vi "3.3-What.vi"() -> ()   [LabVIEW 2010]
uses:
  3.0 Flow Control/3.0 List of Loops.ctl
  4-High Neurons/4.1.2-Act Neuron TD.ctl
  <instrlib>/Hokuyo URG Series/Public/Initialize-Standard.vi
  3.0-Global.vi
  <instrlib>/Hokuyo URG Series/Hokuyo URG Series.lvlib
panel:
  in  "Stop":bool
  out "size(s)":i32
  in  "ID Query?":bool
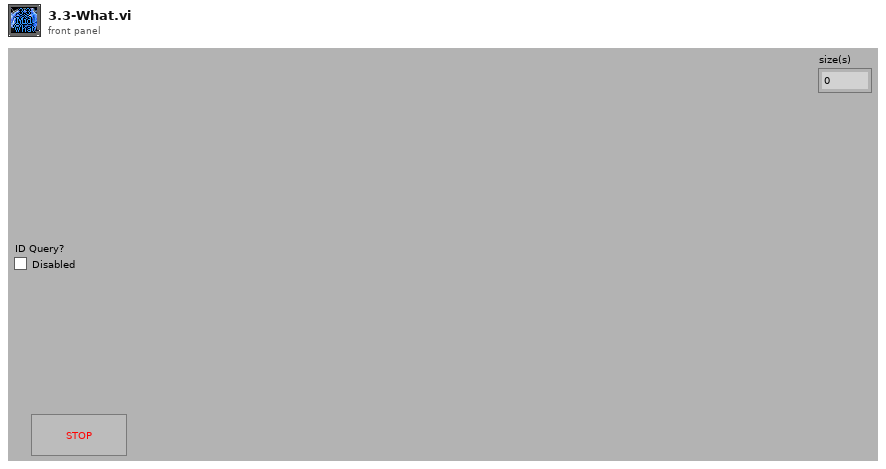
[diagram p1: front panel]
types:
  T1 = typedef "3.0 List of Loops.ctl" = enum16{"3.0 State Update", "3.0 GUI", "3.1 Act", "3.1 4.7.1 Act UDP", "3.1 Joystick", "3.2 Where", "3.2 4.7.2 Where UDP", "3.3 What", "3.3 4.7.3 What UDP", "3.4 How", "3.4 4.7.4 How UDP", "3.5 Limbic", "3.8 TCP", "3.6 Cerebellum"}
  T2 = typedef "4.1.2-Act Neuron TD.ctl" = cluster{"Speed By Path":dbl[]}
  T3 = enum16{"Set Joystick", "Read Joystick", "Set Forebrain", "Read Forebrain", "Set Limbic", "Read Limbic", "Set Cerebellum", "Read Cerebellum", "Set Arbitrated", "Read Arbitrated", "Set LIDAR", "Read LIDAR"}
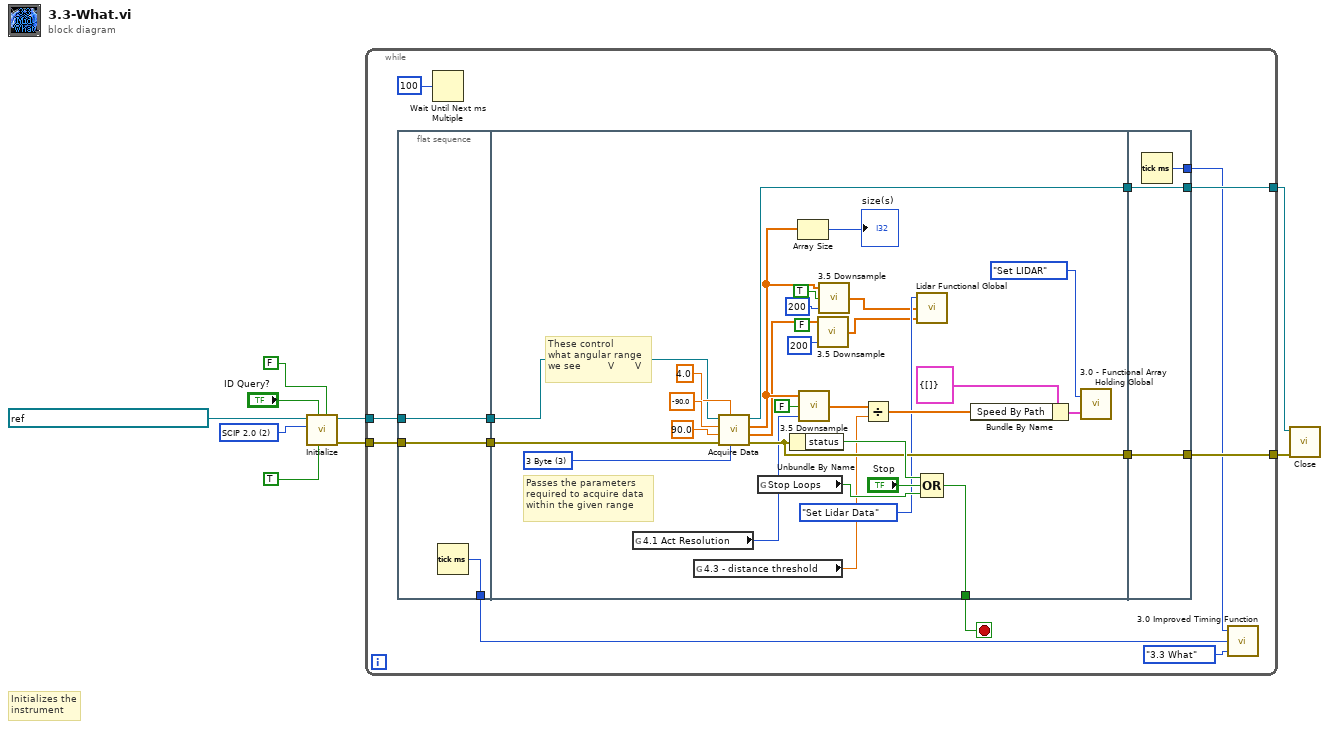
[diagram p0: block diagram]
diagram:
  w2 = u32 2 items=["Convert to Latest", "SCIP 1.1", "SCIP 2.0", "SCIP 2.2"] ("Protocol (2: SCIP 2.0)")
  # "Initializes the instrument"
  n1 = call-poly <instrlib>:"Initialize.vi"("Reset? (F: No)"=FALSE ("Reset Instrument (Disabled)"), "Checksum (Disabled)"=TRUE ("Checksum"), "ID Query? (Enabled)"="ID Query?", "Protocol (2: SCIP 2.0)"=w2, "VISA resource name"=refnum<visa-resource-name> "TCPIP::10.10.10.15::10940::Socket") -> ("error out"=w3:errorcluster, "VISA resource name out"=w4:refnum<visa-resource-name>)  [unwired: 5 in]
  n2 = while {
    tunnel: w4 -> [w21]
    tunnel: [w18] -> w9
    tunnel: [w19] -> w5
    tunnel: w3 -> [w20]
    stop <- w22 stop-if-true
    n3 = flat-sequence {
      tunnel: w20 -> [w24]
      tunnel: w21 -> [w25]
      tunnel: [w25] -> w17
      tunnel: [w24] -> w16
      tunnel: [w23] -> w12
      tunnel: [w52] -> w22
      tunnel: w17 -> [w48]
      tunnel: w16 -> [w47]
      tunnel: [w45] -> w15
      tunnel: [w44] -> w14
      tunnel: [w56] -> w18
      tunnel: [w57] -> w19
      tunnel: w15 -> [w57]
      tunnel: w14 -> [w56]
      tunnel: [w55] -> w13
      frame #0 {
        n4 = Tick Count (ms)() -> (millisecond timer value=w23:u32)
      }
      frame #1 {
        (unwired) FALSE ("Minimum?")
        w46 = u16 3 items=["2 Byte"=2, "3 Byte"=3] ("Encoding Width")
        # "These control\nwhat angular range\nwe see         V       V"
        # "Passes the parameters\nrequired to acquire data\nwithin the given range"
        n5 = global read "3.0-Global.vi" "4.1 Act Resolution"() -> (w38:u32)
        n6 = global read "3.0-Global.vi" "4.3 - distance threshold"() -> (w36:dbl)
        n7 = call <instrlib>:"Acquire Data.vi"("Data Encoding Width (3 Byte)"=w46, "Cluster Count (1)"=4.0 ("Cluster Count"), "error in (no error)"=w47, "End Point (120°)"=90.0 ("End Point"), "Start Point (-120°)"=-90.0 ("Start Point"), "VISA resource name"=w48) -> ("error out"=w44:errorcluster, "Direction"=w30:dbl[], "Magnitude"=w31:dbl[], "VISA resource name out"=w45:refnum<visa-resource-name>)  [unwired: 2 in]
        n8 = global read "3.0-Global.vi" "Stop Loops"() -> (w43:bool)
        n9 = Unbundle By Name(w44) -> ("status"=w54:bool)
        n10 = Array Size(array=w31) -> (size(s)=→"size(s)":i32)
        n11 = call "3.5 Downsample.vi"("Numeric"=w38, "Minimum?"=FALSE, "Input Array"=w31) -> ("Output Array"=w37:sgl[])
        n12 = call "3.5 Downsample.vi"("Numeric"=200, "Input Array"=w30) -> ("Output Array"=w29:sgl[])  [unwired: 1 in]
        n13 = call "3.5 Downsample.vi"("Numeric"=200, "Minimum?"=TRUE, "Input Array"=w31) -> ("Output Array"=w28:sgl[])
        n14 = Divide(x=w37, y=w36) -> (x/y=w35:dbl[])
        n15 = call "Lidar Functional Global.vi"("Lidar Angle Data In (Degrees)"=w29, "Lidar Magnitude Data In (mm)"=w28, "Lidar Action"=enum16{"Set Lidar Data", "Read Lidar Data"}."Set Lidar Data") -> ()  [unwired: 2 out]
        n16 = Compound Arithmetic op=OR(w54, "Stop", w43) -> (w52:bool)
        n17 = Bundle By Name(cluster=T2 {"Speed By Path"=[]} ("Input Act Neurons"), "Speed By Path"=w35) -> (w39:T2)
        n18 = call "3.0 - Functional Array Holding Global.vi"("Input Act Neurons"=w39, "Mode"=T3."Set LIDAR") -> ()  [unwired: 1 out]
      }
      frame #2 {
        n19 = Tick Count (ms)() -> (millisecond timer value=w55:u32)
      }
    }
    n20 = Wait Until Next ms Multiple(millisecond multiple=u32 100) -> ()  [unwired: 1 out]
    n21 = call "3.0 Improved Timing Function.vi"("Loop"=3.0_List_of_Loops."3.3 What", "Start"=w12, "End"=w13) -> ()  [unwired: 1 in]
  }
  n22 = call <instrlib>:"Close.vi"("error in (no error)"=w9, "VISA resource name"=w5) -> ()  [unwired: 9 in, 1 out]
